vi "FTW-Connector-SendPoisonPill.vi"(0 "FTW Actor Connector":refnum<class "FTW-Actor-Connector.lvclass">, 5 "Timeout":i32=500 format="%dmsec", 11 "error in":errorcluster) -> (4 "FTW Actor Connector out":refnum<class "FTW-Actor-Connector.lvclass">, 6 "Response":string, 8 "Timed out?":bool, 15 "error out":errorcluster)   [LabVIEW 2013, in "FTW-Actor-Connector.lvclass"]
uses:
  FTW-Actor-Connector.lvclass
panel:
  # "Inputs"
  # "Outputs"
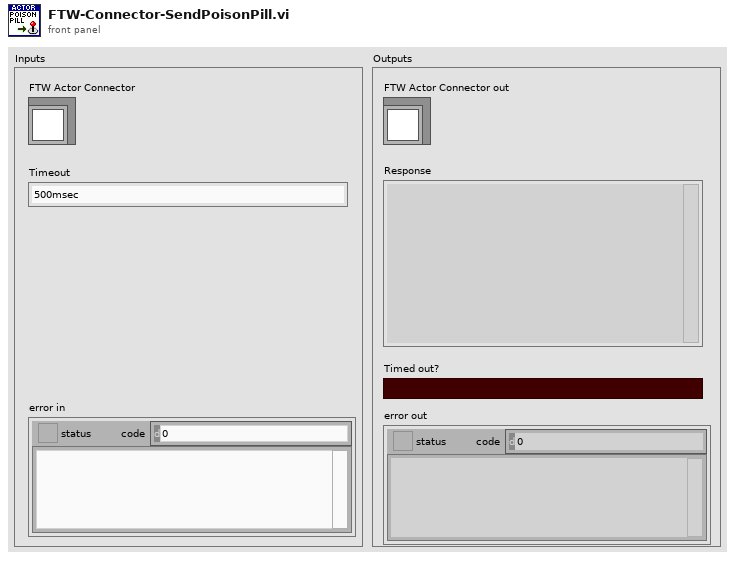
[diagram p1: front panel]
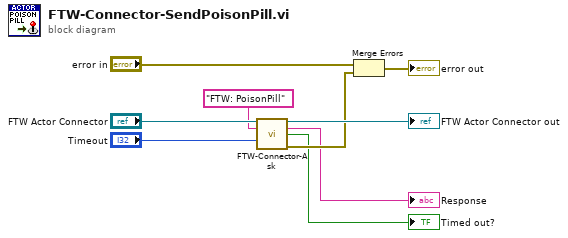
[diagram p0: block diagram]
diagram:
  n1 = call "FTW-Connector-Ask.vi"("FTW Actor Connector"="FTW Actor Connector", "Request Header"="FTW: PoisonPill" ("Message"), "Timeout"="Timeout") -> ("FTW Actor Connector out"=→"FTW Actor Connector out":refnum<class "FTW-Actor-Connector.lvclass">, "Response Body"=→"Response":string, "Timed out?"=→"Timed out?":bool, "error out"=w4:errorcluster)  [unwired: 9 in]
  n2 = Merge Errors("error in", w4) -> (→"error out":errorcluster)
